vi "Wire Probe.vi"(11 "channel":T1) -> (2 "Value String":string="See Channel Status Window for information.", 3 "Boolean":bool)   [LabVIEW 2019, in "MessengerM.lvlib"]
uses:
  <resource>/Channels/MessengerM/MessengerM.lvlib
  <resource>/Channels/MessengerM/ChannelOp.ctl
  <resource>/Channels/MessengerM/MessengerMCPU/MessengerMCPU.lvclass
  Applications/National Instruments/LabVIEW 2019 64-bit/resource/Channels/MessengerM/MessengerMBase/MessengerMBase.lvclass
  <resource>/Channels/MessengerM/))Channel.ctl
  <resource>/Channels/MessengerM/Element.ctl
panel:
  in  "Default Text":string="* If the diagram containing this channel wire has already activated, the channel probe will open immediately.\n\n* Otherwise, the channel probe will open when the diagram that contains this wire probe next activates. To probe a channel from the very beginning of its lifetime, set a wire probe on the channel wire at the highest level diagram where branches from the writers and readers meet up. See \"Probing Channel Wires\" in the LabVIEW help for more information."
  out "Display":string="* If the diagram containing this channel wire has already activated, the channel probe will open immediately.\n\n* Otherwise, the channel probe will open when the diagram that contains this wire probe next activates. To probe a channel from the very beginning of its lifetime, set a wire probe on the channel wire at the highest level diagram where branches from the writers and readers meet up. See \"Probing Channel Wires\" in the LabVIEW help for more information."
  in  "pause on activation?":bool
  in  "Could Not Allocate Probe":string="Could not create probe because of low memory. Please free up memory so that LabVIEW may allocate a channel probe."
  in  "Mismatched Type":string="Could not create probe because of type mismatch. Please alert National Instruments about this error. Until this is repaired, channels of this kind cannot be probed."
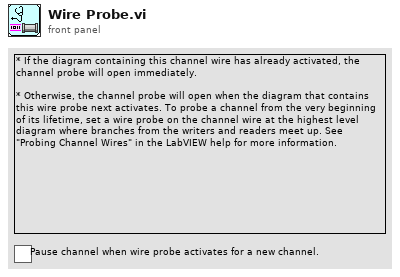
[diagram p1: front panel]
types:
  T1 = typedef "MessengerM.lvlib/))Channel.ctl" = refnum<queue>
  T2 = typedef "MessengerM.lvlib/ChannelOp.ctl" = enum16{"init", "write", "read", "wreplace", "rreplace", "wrtAck", "rdAck", "rdAck2", "packet", "probe"}
  T3 = enum32{"Invalid", "Standard", "Closed", "Hidden", "Minimized", "Maximized"}
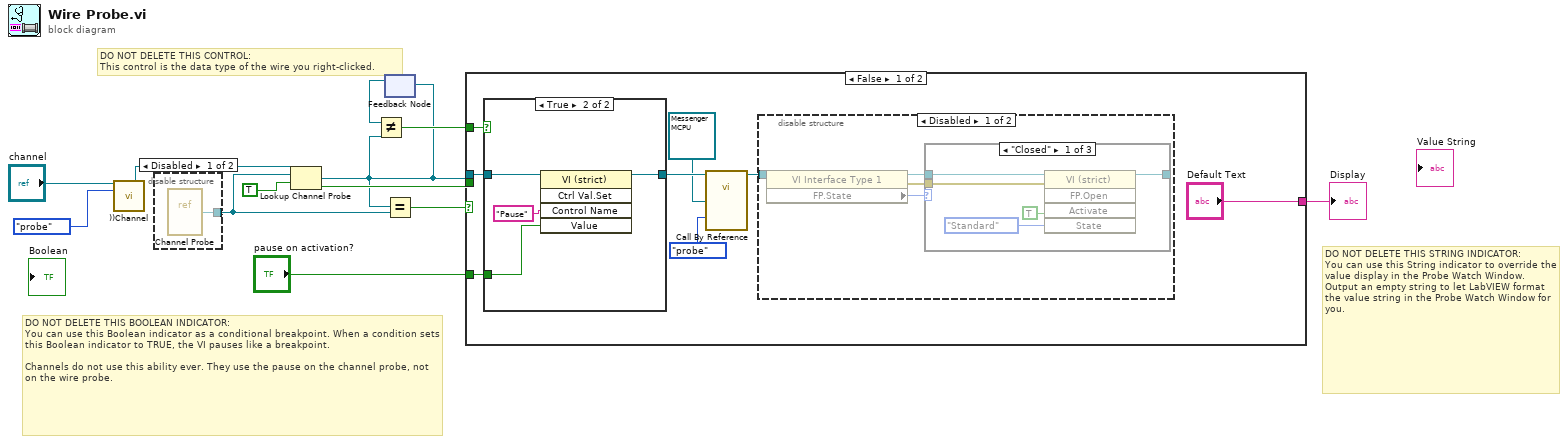
[diagram p0: block diagram]
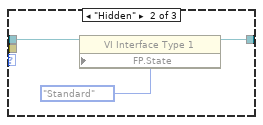
[diagram p3: hidden frame]
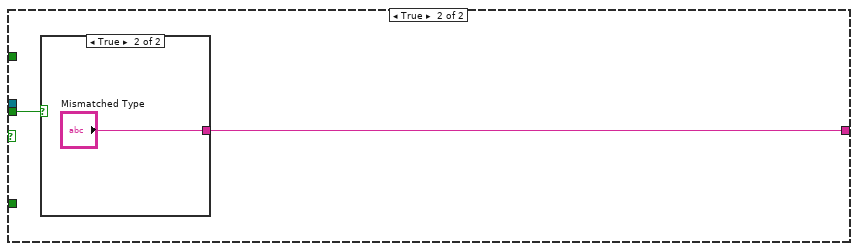
[diagram p7: hidden frame]
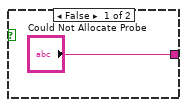
[diagram p8: hidden frame]
diagram:
  # "DO NOT DELETE THIS STRING INDICATOR: \nYou can use this String indicator to override the value display in the Probe Watch Window.  Output an empty string to let LabVIEW format the value string in the Probe Watch Window for you."
  # "DO NOT DELETE THIS BOOLEAN INDICATOR: \nYou can use this Boolean indicator as a conditional breakpoint. When a condition sets this Boolean indicator to TRUE, the VI pauses like a breakpoint.\n\nChannels do not use this ability ever. They use the pause on the channel probe, not on the wire probe."
  # "DO NOT DELETE THIS CONTROL: \nThis control is the data type of the wire you right-clicked."
  n1 = call <resource>:"))Channel.vi"("channel in"="channel", "channelOp"=ChannelOp."probe") -> ("This VI out"=w1:refnum<vi>)  [unwired: 8 in, 5 out]
  n2 = disable-structure shown="Disabled" {
    disable-tunnel: [w13 _] -> w2
    frame Disabled {
      n3 = vi-ref <resource>:"Channel Probe.vi"() -> (w13:refnum<vi>)
    }
    frame Enabled {
    }
  }
  n4 = Lookup Channel Probe(0:w1, 1:w2, 2:TRUE ("force create?")) -> (9:w6:refnum<vi>, 10:w10:bool)
  n5 = feedback-in #1(w6) -> ()
  n6 = feedback #1() -> (w8:refnum<vi>)  [unwired: 1 in]
  n7 = Not Equal?(x=w8, y=w6) -> (x != y?=w7:bool)
  n8 = Equal?(x=w6, y=w2) -> (x = y?=w11:bool)
  n9 = case shown="False" w11 {
    tunnel: w10 -> [_ w41]
    tunnel: ["Default Text" w40] -> w5
    tunnel: w6 -> [w21 _]
    tunnel: "pause on activation?" -> [w20 _]
    tunnel: w7 -> [w19 _]
    frame False {
      n10 = case shown="True" w19 {
        tunnel: w21 -> [w35 w39]
        tunnel: w20 -> [_ w37]
        tunnel: [w35 w36] -> w18
        frame False {
        }
        frame True {
          n11 = invoke class="VI (strict)" method="Ctrl Val.Set"(reference=w39, "Control Name"="Pause", "Value"=w37) -> (reference out=w36:refnum<vi>)  [unwired: 2 in, 4 out]
        }
      }
      n12 = call-by-ref "?"(reference=w18, "channelOp"=ChannelOp."probe", "mdata in"=refnum<class "MessengerMCPU.lvclass"> refnum) -> (reference out=w17:refnum<vi>)  [unwired: 2 in, 2 out]
      n13 = disable-structure shown="Disabled" {
        disable-tunnel: w17 -> [w22 _]
        frame Disabled {
          n14 = property class="VI Interface Type 1"(reference=w22) -> (reference out=w23:refnum<vi>, error out=w24:errorcluster, "FP.State"=w25:T3)  [unwired: 1 in]
          n15 = case shown="\"Closed\"" w25 {
            tunnel: w24 -> [w29 _ _]
            tunnel: w23 -> [w30 w33 w34]
            tunnel: [w26 w32 w34] -> _
            frame "Closed" {
              n16 = invoke class="VI (strict)" method="FP.Open"(reference=w30, error in=w29, "Activate"=TRUE ("Activate?"), "State"=T3."Standard") -> (reference out=w26:refnum<vi>)  [unwired: 1 in, 4 out]
            }
            frame "Hidden" {
              n17 = property class="VI Interface Type 1"(reference=w33, "FP.State"=T3."Standard" ("Front Panel Window:State")) -> (reference out=w32:refnum<vi>)  [unwired: 1 in, 1 out]
            }
            frame Default {
            }
          }
        }
        frame Enabled {
        }
      }
    }
    frame True {
      n18 = case shown="True" w41 {
        tunnel: ["Could Not Allocate Probe" "Mismatched Type"] -> w40
        frame False {
        }
        frame True {
        }
      }
    }
  }
  "Display" <- w5
